vi "test_Find FPGA Addons.vi"(8 "error in (no error)":errorcluster, 11 "TestCase in":refnum<class "FPGA Addon Scripting API Unit Tests.lvclass">) -> (0 "error out":errorcluster, 3 "TestCase out":refnum<class "FPGA Addon Scripting API Unit Tests.lvclass">)   [LabVIEW 2020, in "FPGA Addon Scripting API Unit Tests.lvclass"]
uses:
  FPGA Addon Scripting API Unit Tests.lvclass
  <vilib>/addons/_JKI Toolkits/VI Tester/TestCase.llb/TestCase.lvclass
  FPGA Addon Test Class/FPGA Addon Test Class.lvclass
  <vilib>/NI VeriStand/Custom Device Tools/Custom Device Utility Library/Custom Device Utility Library.lvlib
  APIs/Scripting API/Scripting API.lvlib
  C:/Program Files (x86)/National Instruments/LabVIEW 2020/vi.lib/addons/_JKI Toolkits/VI Tester/TestCase.llb/TestCase.lvclass
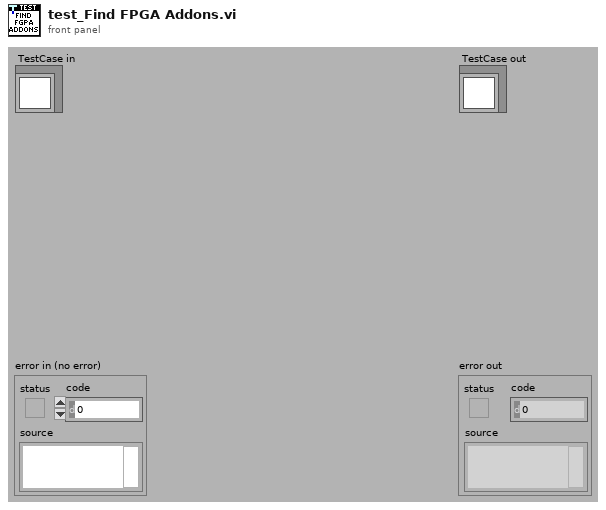
[diagram p1: front panel]
types:
  T1 = typedef "Custom Device API.lvlib/Custom Device Item Ref.ctl" = u64
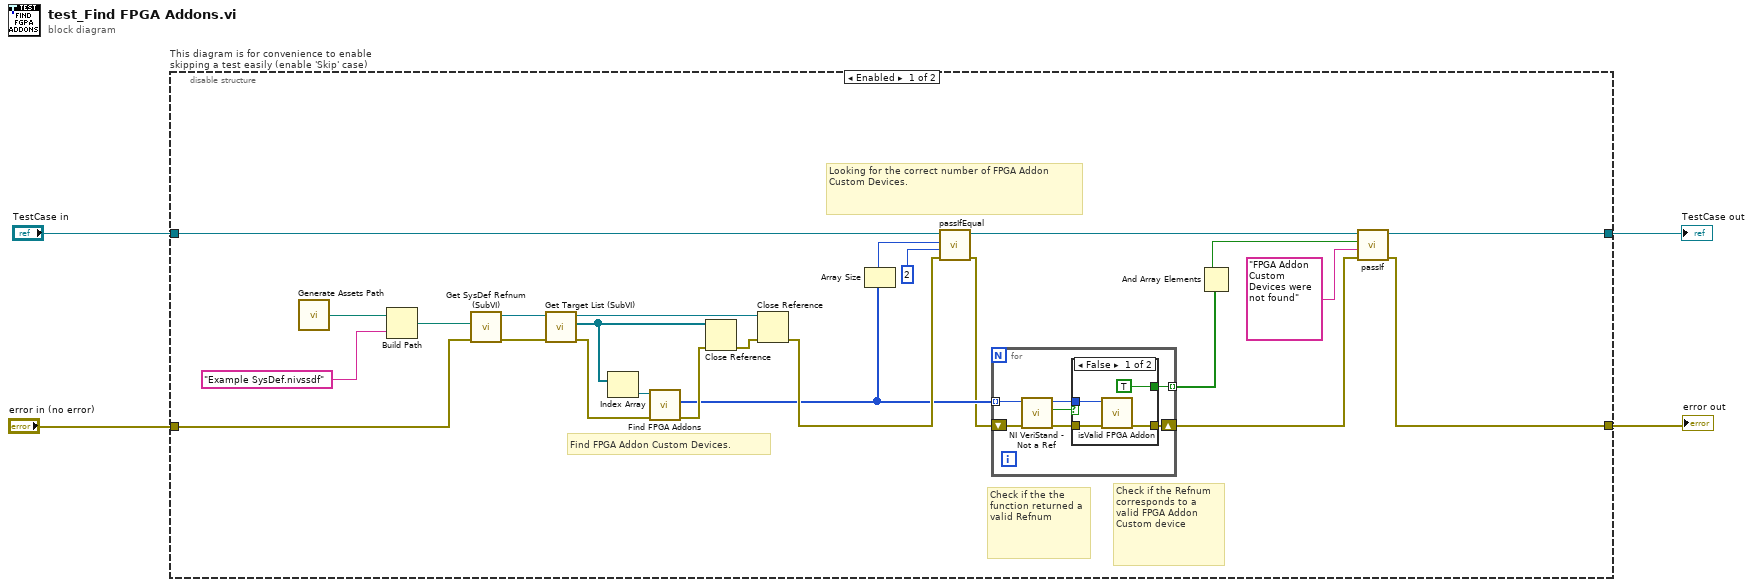
[diagram p0: block diagram]
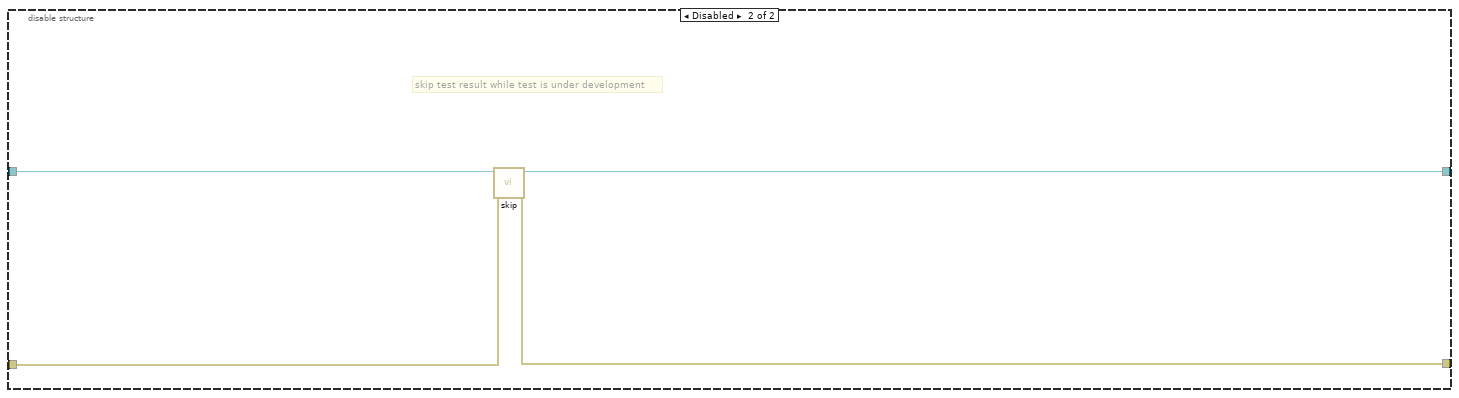
[diagram p3: hidden frame]
diagram:
  n1 = disable-structure "This diagram is for convenience to enable skipping a test easily (enable 'Skip' case)" shown="Enabled" {
    disable-tunnel: "TestCase in" -> [w11 w45]
    disable-tunnel: [w18 w43] -> w1
    disable-tunnel: [w17 w44] -> w3
    disable-tunnel: "error in (no error)" -> [w25 w42]
    frame Enabled {
      # "Find FPGA Addon Custom Devices."
      # "Check if the Refnum corresponds to a valid FPGA Addon Custom device"
      # "Check if the the function returned a valid Refnum"
      # "Looking for the correct number of FPGA Addon Custom Devices."
      n2 = call "Generate Assets Path.vi"() -> ("Assets path"=w29:path)
      n3 = Build Path(base path=w29, name or relative path="Example SysDef.nivssdf") -> (appended path=w27:path)
      n4 = call "Get SysDef Refnum (SubVI).vi"("error in (no error)"=w25, "System Definition path"=w27) -> ("error out"=w24:errorcluster, "SysDef Refnum out"=w26:refnum<k24>)  [unwired: 8 in]
      n5 = call "Get Target List (SubVI).vi"("error in (no error)"=w24, "SysDef Refnum in"=w26) -> ("error out"=w15:errorcluster, "Target List Refnums"=w22:refnum<k24>[], "SysDef Refnum out"=w21:refnum<k24>)  [unwired: 7 in]
      n6 = Index Array(array=w22) -> (element=w16:refnum<k24>)  [unwired: 1 in]
      n7 = call "Find FPGA Addons.vi"("error in"=w15, "target in"=w16) -> ("error out"=w14:errorcluster, "FPGA addon refnums out"=w9:T1[])  [unwired: 6 in, 2 out]
      n8 = Close Reference(reference=w22, error in (no error)=w14) -> (error out=w20:errorcluster)
      n9 = Close Reference(reference=w21, error in (no error)=w20) -> (error out=w10:errorcluster)
      n10 = Array Size(array=w9) -> (size(s)=w8:i32)
      n11 = call-dynamic "passIfEqual.vi"("error in (no error)"=w10, "y"=2 ("size(s)"), "x"=w8, "TestCase in"=w11) -> ("error out"=w5:errorcluster, "TestCase out"=w6:refnum<class "FPGA Addon Scripting API Unit Tests.lvclass">)  [unwired: 6 in]
      n12 = for {
        shift-right: [w33] -> w19
        shift-left: w5 -> [w36]
        tunnel: w9 -> [w31] mode=indexing
        tunnel: [w30] -> w13 mode=indexing
        n13 = call <vilib>:"NI VeriStand - Not a Ref.vi"("error in (no error)"=w36, "Item Ref"=w31) -> ("error out"=w34:errorcluster, "Not a Ref"=w32:bool, "Item Ref out"=w35:T1)  [unwired: 7 in]
        n14 = case shown="False" w32 {
          tunnel: w35 -> [w40 _]
          tunnel: w34 -> [w39 w41]
          tunnel: [w38 w41] -> w33
          tunnel: [TRUE _] -> w30
          frame False {
            n15 = call "isValid FPGA Addon.vi"("error in"=w39, "FPGA Addon refnum in"=w40) -> ("error out"=w38:errorcluster)  [unwired: 8 in, 1 out]
          }
          frame True {
          }
        }
      }
      n16 = And Array Elements(Boolean array=w13) -> (logical AND=w12:bool)
      n17 = call-dynamic "passIf.vi"("error in (no error)"=w19, "message (\"\")"="FPGA Addon Custom Devices were not found" ("message (\"\")"), "pass"=w12, "TestCase in"=w6) -> ("error out"=w17:errorcluster, "TestCase out"=w18:refnum<class "FPGA Addon Scripting API Unit Tests.lvclass">)  [unwired: 6 in]
    }
    frame Disabled {
      # "skip test result while test is under development"
      n18 = call <vilib>:"skip.vi"("error in (no error)"=w42, "TestCase in"=w45) -> ("error out"=w44:errorcluster, "TestCase out"=w43:refnum<class "FPGA Addon Scripting API Unit Tests.lvclass">)  [unwired: 8 in]
    }
  }
  "error out" <- w3
  "TestCase out" <- w1
